vi "生成任务队列.vi"(11 "循环次数":u32) -> (3 "数组":string[](array[string]))   [LabVIEW 2021]
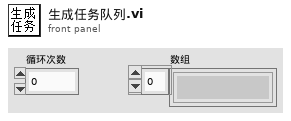
[diagram p1: front panel]
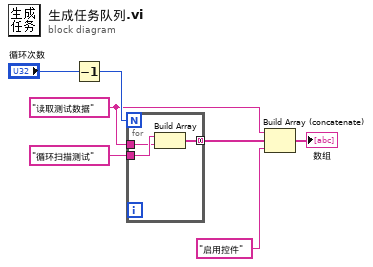
[diagram p0: block diagram]
diagram:
  w2 = "读取测试数据" ("消息")
  n1 = Decrement(x="循环次数") -> (x-1=w7:u32)
  n2 = for {
    N: w7 -> [_]
    tunnel: "循环扫描测试" ("消息") -> [w10]
    tunnel: w2 -> [w9]
    tunnel: [w8] -> w3 mode=concatenating
    n3 = Build Array(w10, w9) -> (w8:string[])
  }
  n4 = Build Array (concatenate)(w2, w3, "启用控件" ("元素")) -> (→"数组":string[])
